vi "AlliGator SNIAL Abort.vi"() -> ()   [LabVIEW 2021, in "AlliGator Shot Noise Influence on Average Lifetime.lvlib"]
doc: "Used to interrupt tasks in scripts."
uses:
  AlliGator Shot Noise Influence on Average Lifetime.lvlib
panel:
  out "Abort?":bool
  # "see the AlliGator License on the block diagram (Ctrl+E or Window:Show Block Diagram)"
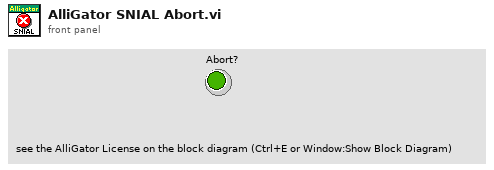
[diagram p1: front panel]
diagram:
